vi "Shape.vi"(7 "chips":cdb[](array[numeric])) -> (8 "envelope":cdb[](array[numeric]))   [LabVIEW 2017]
uses:
  <vilib>/addons/Modulation/Analog/support/mod_Set Error Source.vi
  <vilib>/addons/Modulation/Digital/Support/Common/Validators/mod_Generate Filter Coefficients Validate.vi
  <vilib>/addons/Modulation/Digital/General/subVIs/mod_Generate Filter Coefficients.vi
  <vilib>/Analysis/2dsp.llb/Upsample (CDB).vi
  <vilib>/Analysis/3filter.llb/FIR Filter (CDB).vi
  <vilib>/addons/Modulation/niDMT.lvlib
  <vilib>/Analysis/NI_AALBase.lvlib
  <vilib>/Analysis/NI_AALPro.lvlib
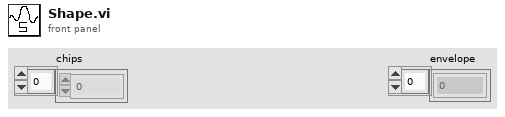
[diagram p1: front panel]
types:
  T1 = enum16{"none", "Raised Cosine", "Root Raised Cos", "Gaussian"}
  T2 = enum16{"FSK", "PSK", "QAM", "MSK", "PAM", "ASK", "CPM"}
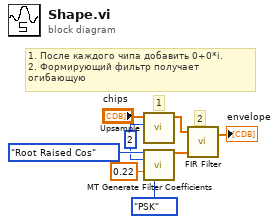
[diagram p0: block diagram]
diagram:
  w3 = 2 ("upsampling factor")
  # "1. После каждого чипа добавить 0+0*i.\n2. Формирующий фильтр получает\nогибающую"
  # "2"
  # "1"
  n1 = call-poly <vilib>:"Upsample.vi"("upsampling factor"=w3, "X"="chips") -> ("Upsampled Array"=w4:cdb[])  [unwired: 8 in, 1 out]
  n2 = call <vilib>:"MT Generate Filter Coefficients.vi"("pulse shaping filter (none)"=T1."Root Raised Cos", "modulation type"=T2."PSK", "pulse shaping samples per symbol (16)"=w3, "filter parameter"=0.22) -> ("pulse shaping filter coefficients"=w5:dbl[])  [unwired: 9 in, 2 out]
  n3 = call-poly <vilib>:"FIR Filter.vi"("FIR Coefficients"=w5, "X"=w4) -> ("Filtered X"=→"envelope":cdb[])  [unwired: 2 in, 1 out]
